vi "Test_Copy_Image_ARGB_Mask_ARGB.vi"(8 "error in (no error)":errorcluster, 11 "Test Case In":refnum<class "Image.lvclass">) -> (0 "error out":errorcluster, 3 "Test Case Out":refnum<class "Image.lvclass">)   [LabVIEW 2020, in "g_ar_toolkit.test.lvlib" / "Image.lvclass"]
uses:
  Image.lvclass
  Image.lvclass/Image.ctl
  g_ar_toolkit.image/g_ar_toolkit.image.lvlib
  g_ar_toolkit.image/Image Size (Fixed).ctl
  g_ar_toolkit.image/CreateEmptyImageARGB.vi
  g_ar_toolkit.image/CopyImageARGBMaskARGB.vi
  g_ar_toolkit.image/ARGB Colour.ctl
  4993e8ee-a06a-463a-9684-69129f64d5ce.vi
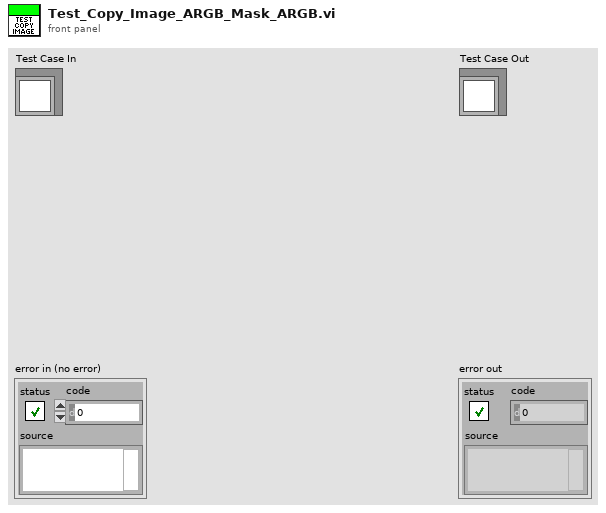
[diagram p1: front panel]
types:
  T1 = typedef "g_ar_toolkit.image.lvlib/ARGB Colour.ctl" = cluster{"Alpha":u8, "RGB":u32}
  T2 = typedef "g_ar_toolkit.image.lvlib/Image Size (Fixed).ctl" = cluster{"Width":u16, "Height":u16}
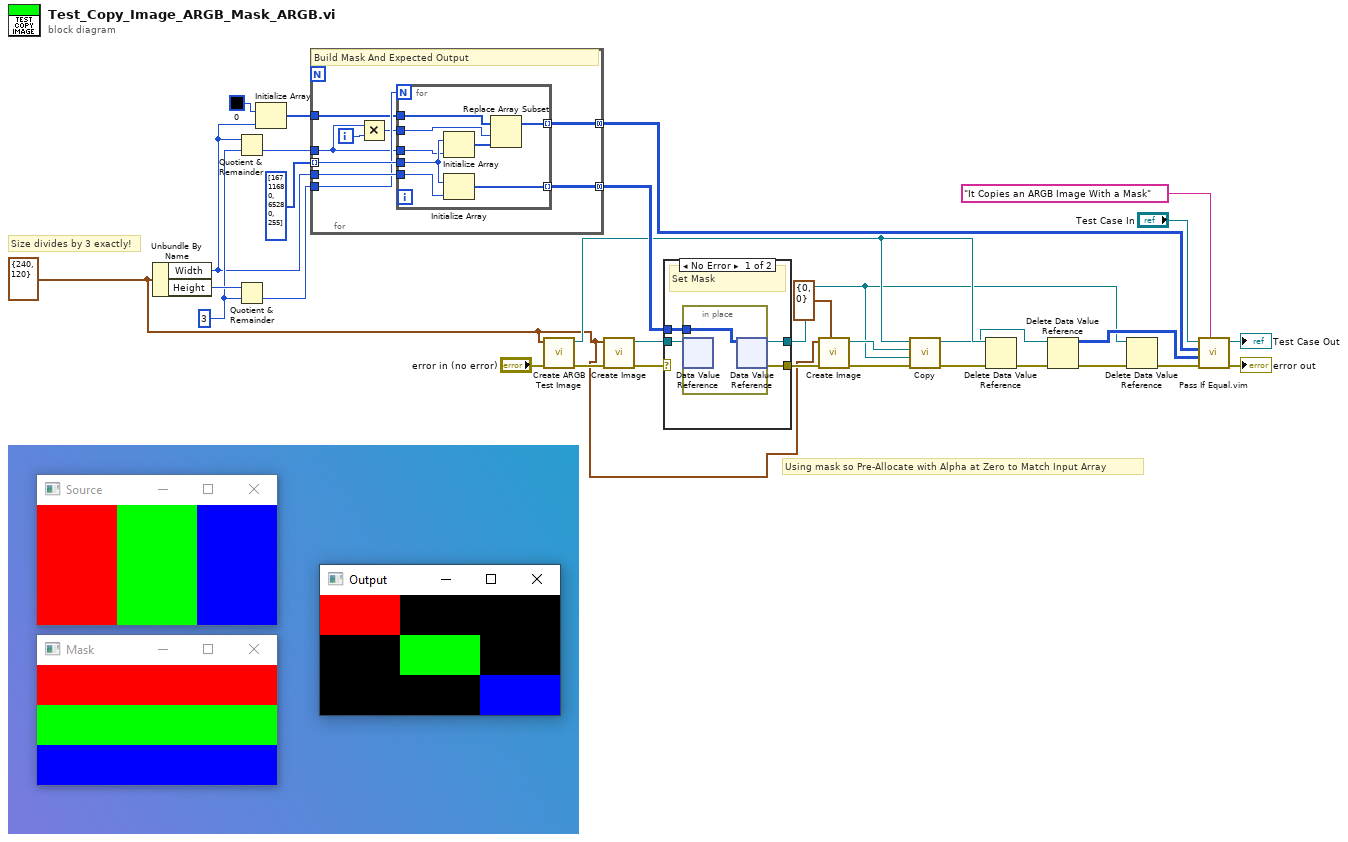
[diagram p0: block diagram]
diagram:
  w17 = u16 3 ("y")
  w1 = T2 {"Width"=240, "Height"=120} ("Preallocated Image Size (Default - 0,0)")
  # "Using mask so Pre-Allocate with Alpha at Zero to Match Input Array"
  # "Size divides by 3 exactly!"
  n1 = Unbundle By Name(w1) -> ("Width"=w15:u16, "Height"=w24:u16)
  n2 = Quotient & Remainder(x=w15, y=w17) -> (floor(x/y)=w16:u16)  [unwired: 1 out]
  n3 = Quotient & Remainder(x=w24, y=w17) -> (floor(x/y)=w23:u16)  [unwired: 1 out]
  n4 = Initialize Array(u32 0, w15) -> (w13:u32[])
  n5 = for {
    tunnel: u32[] [16711680, 65280, 255] ("color(black)") -> [w40] mode=indexing
    tunnel: w15 -> [w39]
    tunnel: [w38] -> w22 mode=concatenating
    tunnel: w23 -> [w37]
    tunnel: w16 -> [w33]
    tunnel: w13 -> [w34]
    tunnel: [w32] -> w12 mode=concatenating
    i -> [w36]
    # "Build Mask And Expected Output"
    n6 = Multiply(x=w33, y=w36) -> (x*y=w35:i32)
    n7 = for {
      N: w37 -> [_]
      tunnel: w40 -> [w46]
      tunnel: w39 -> [w48]
      tunnel: [w47] -> w38 mode=indexing
      tunnel: w35 -> [w42]
      tunnel: w34 -> [w44]
      tunnel: w33 -> [w45]
      tunnel: [w41] -> w32 mode=indexing
      n8 = Initialize Array(w46, w45) -> (w43:u32[])
      n9 = Initialize Array(w46, w48) -> (w47:u32[])
      n10 = Replace Array Subset(array=w44, new element=w43, index=w42) -> (w41:u32[])
    }
  }
  n11 = call "Create ARGB Test Image.vi"("error in (no error)"="error in (no error)", "Preallocated Image Size"=w1) -> ("error out"=w10:errorcluster, "Data Value Reference out"=w7:refnum<data-value>)  [unwired: 7 in, 1 out]
  n12 = call-poly "Create Image.vi"("error in (no error)"=w10, "Preallocated Image Size (Default: 0,0)"=w1) -> ("error out"=w20:errorcluster, "New ARGB Image"=w21:refnum<data-value>)  [unwired: 8 in]
  n13 = case shown="No Error" w20 {
    selector: w20 -> [_ w54]
    tunnel: w21 -> [w52 w55]
    tunnel: [w51 w55] -> w4
    tunnel: [w50 w54] -> w19
    tunnel: w22 -> [w49 _]
    frame No Error {
      # "Set Mask"
      n14 = in-place {
        in-place-border: w49 -> [w53]
        n15 = in-place-dvr #1(w52) -> ()  [unwired: 2 out]
        n16 = in-place-dvr #1(w53) -> (w51:refnum<data-value>, w50:errorcluster)
      }
    }
    frame Error {
    }
  }
  n17 = call-poly "Create Image.vi"("Colour (Default: Black)"=T1 {"Alpha"=0, "RGB"=0}, "error in (no error)"=w19, "Preallocated Image Size (Default: 0,0)"=w1) -> ("error out"=w27:errorcluster, "New ARGB Image"=w9:refnum<data-value>)  [unwired: 7 in]
  n18 = call-poly "Copy.vi"("error in (no error)"=w27, "ARGB Image Mask"=w4, "ARGB Image Destination"=w9, "ARGB Image Source"=w7) -> ("error out"=w8:errorcluster, "ARGB Image Destination (duplicate)"=w6:refnum<data-value>)  [unwired: 6 in]
  n19 = Delete Data Value Reference(data value reference=w7, error in=w8) -> (error out=w18:errorcluster)  [unwired: 1 out]
  n20 = Delete Data Value Reference(data value reference=w6, error in=w18) -> (data value=w26:u32[][], error out=w5:errorcluster)
  n21 = Delete Data Value Reference(data value reference=w4, error in=w5) -> (error out=w3:errorcluster)  [unwired: 1 out]
  n22 = call "Pass If Equal.vim"("Description"="It Copies an ARGB Image With a Mask", "error in (no error)"=w3, "Actual"=w26, "Expected"=w12, "LUnit Test Case In"="Test Case In") -> ("error out"=→"error out":errorcluster, "LUnit Test Case Out"=→"Test Case Out":refnum<class "Image.lvclass">)  [unwired: 5 in]
